vi "Do.vi"(8 "error in (no error)":errorcluster, 10 "Actor in":refnum<class "Actor.lvclass">, 11 "Send Change Frequency MSG":refnum<class "Send Change Frequency MSG.lvclass">) -> (0 "error out":errorcluster, 2 "Actor out":refnum<class "Actor.lvclass">)   [LabVIEW 2014, in "Controller.lvlib" / "Send Change Frequency MSG.lvclass"]
doc: "(<B>Filename</B>: Actor Framework.lvlib:Message.lvclass:Do.vi)\n\nDefines what a message does when it is received by an actor. Generally, a message instructs an actor to invoke one of its methods. By default, this method does nothing. A child class must override it to define behavior. Create a child class by using the Actor Framework Message Maker dialog box."
uses:
  Send Change Frequency MSG.lvclass
  <vilib>/ActorFramework/Actor/Actor.lvclass
  Send Change Frequency MSG.lvclass/Send Change Frequency MSG.ctl
  Calibration/O3 Frequency Train Actor/Messages/Change Frequency MSG/Change Frequency MSG.lvclass
  <vilib>/ActorFramework/Message Enqueuer/Message Enqueuer.lvclass
  Controller.lvclass
  Controller.lvclass/Controller.ctl
  Calibration/O3 Frequency Train Actor/Messages/Change Frequency MSG/Change Frequency MSG.lvclass/Change Frequency MSG.ctl
  <vilib>/ActorFramework/Message Enqueuer/Message Enqueuer.lvclass/Message Enqueuer.ctl
  Calibration/O3 Frequency Train Actor/Messages/Change Frequency MSG/Write freq.vi
  Accessors/Read Enqueuer Map.vi
  <vilib>/ActorFramework/Message Priority Queue/Priority Enqueue.vi
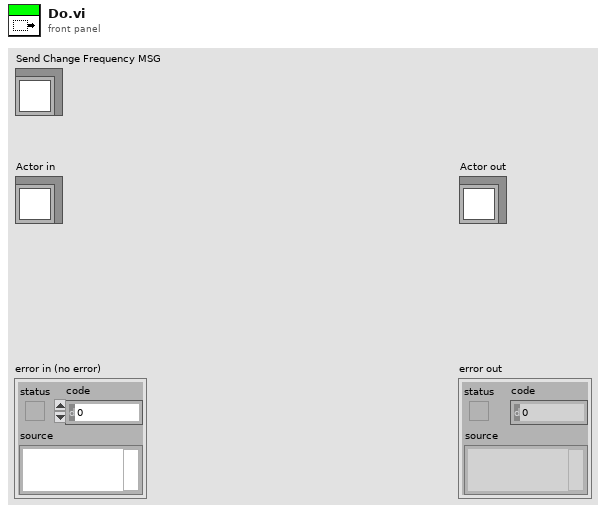
[diagram p1: front panel]
types:
  T1 = cluster{"Message Enqueuer out":refnum<class "Message Enqueuer.lvclass">, bool}
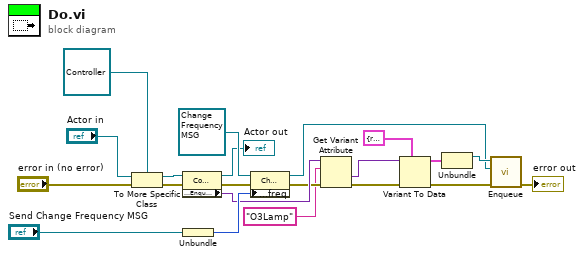
[diagram p0: block diagram]
diagram:
  n1 = To More Specific Class(target class=refnum<class "Controller.lvclass"> refnum ("Controller:Controller"), reference="Actor in", error in="error in (no error)") -> (specific class reference=w11:refnum<class "Controller.lvclass">, error out=w6:errorcluster)
  n2 = property class="Controller"(reference=w11, error in=w6) -> (reference out=→"Actor out":refnum<class "Controller.lvclass">, error out=w5:errorcluster, "Accessors:Enqueuer Map"=w10:variant)
  n3 = Unbundle("Send Change Frequency MSG") -> (w18:i64)
  n4 = property class="Change Frequency MSG.lvclass"(reference=refnum<class "Change Frequency MSG.lvclass"> refnum ("Calibration.lvlib:Change Frequency MSG.lvclass"), error in=w5, "Accessors:freq"=w18) -> (reference out=w1:refnum<class "Change Frequency MSG.lvclass">, error out=w9:errorcluster)
  n5 = Get Variant Attribute(Variant=w10, name="O3Lamp" ("format string"), error in=w9) -> (value=w16:variant, error out=w3:errorcluster)  [unwired: 1 in, 2 out]
  n6 = Variant To Data(error in=w3, type=T1 {"Message Enqueuer out"=refnum, TRUE}, Variant=w16) -> (data=w14:T1, error out=w2:errorcluster)
  n7 = Unbundle(w14) -> ("Message Enqueuer out"=w13:refnum<class "Message Enqueuer.lvclass">)  [unwired: 1 out]
  n8 = call <vilib>:"Enqueue.vi"("error in (no error)"=w2, "Message"=w1, "Message Enqueuer in"=w13) -> ("error out"=→"error out":errorcluster)  [unwired: 7 in, 1 out]
